vi "Auto Axis Align.vi"(9 "Yaw":dbl, 10 "Base Speed":dbl, 11 "Correction Factor":dbl) -> (2 "Right":dbl, 3 "Left":dbl)   [LabVIEW 2016]
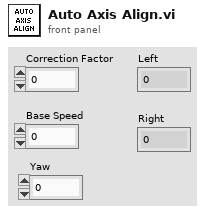
[diagram p1: front panel]
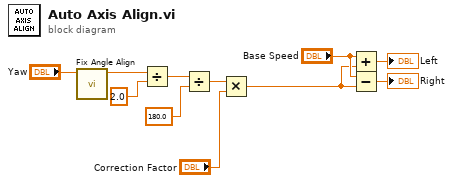
[diagram p0: block diagram]
diagram:
  n1 = call "Fix Angle Align.vi"("Right Setpoint"="Yaw") -> ("Fixed Angle"=w3:dbl)  [unwired: 10 in]
  n2 = Divide(x=w3, y=2.0) -> (x/y=w7:dbl)
  n3 = Divide(x=w7, y=180.0) -> (x/y=w5:dbl)
  n4 = Multiply(x=w5, y="Correction Factor") -> (x*y=w1:dbl)
  n5 = Add(x="Base Speed", y=w1) -> (x+y=→"Left":dbl)
  n6 = Subtract(x="Base Speed", y=w1) -> (x-y=→"Right":dbl)
